vi "CreateQbus.vi"(8 "error in (no error)":errorcluster) -> (0 "error out":errorcluster, 3 "Qbus":refnum<class "Qbus.lvclass">)   [LabVIEW 2017, in "Qbus.lvclass"]
doc: "Initializes the Qbus message bus and returns a reference that integrates other processes with Qbus. Ensure this VI runs before you create Qbus listeners for any processes in the device software."
uses:
  <vilib>/addons/Qbus/Qbus.lvclass
  <vilib>/addons/Qbus/controls/data.ctl
  <vilib>/addons/Qbus/Qbus.lvclass/Qbus.ctl
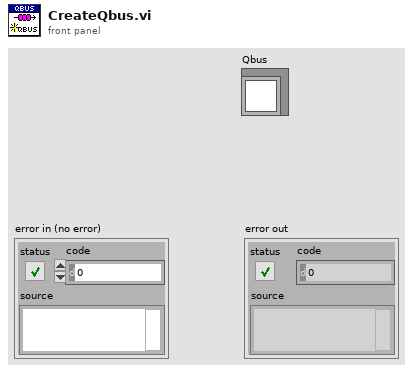
[diagram p1: front panel]
types:
  T1 = typedef "Qbus.lvclass/data.ctl" = cluster{"Queues":variant, "Subscriptions":variant, "MasterQ":string}
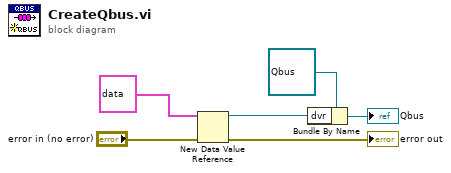
[diagram p0: block diagram]
diagram:
  n1 = New Data Value Reference(data value=T1 {"Queues"=variant, "Subscriptions"=variant, "MasterQ"=""} ("data"), error in="error in (no error)") -> (data value reference=w3:refnum<data-value>, error out=→"error out":errorcluster)
  n2 = Bundle By Name(cluster=refnum<class "Qbus.lvclass"> refnum ("Qbus"), "dvr"=w3) -> (→"Qbus":refnum<class "Qbus.lvclass">)
